vi "lorenz system.vi"(9 "Numeric":i32, 10 "array":dbl[](array[numeric])) -> (1 "z":dbl[](array[numeric]), 2 "y":dbl[](array[numeric]), 3 "x":dbl[](array[numeric]))   [LabVIEW 2019]
uses:
  <vilib>/Native 3D Graph/xcontrol/3DPC_SurfacePlot.xctl
panel:
  out "3D Graph":refnum<class "Base Datatype.lvclass">[](xcontrol)
  # "10*(y - x)\n x*(28 - z) - y\n x*y - (8/3)*z"
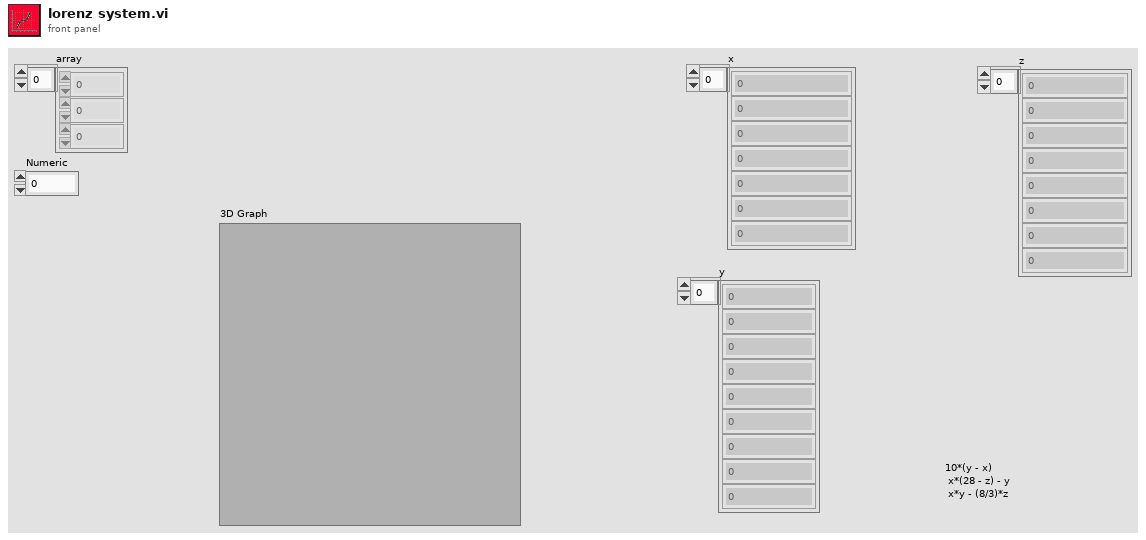
[diagram p1: front panel]
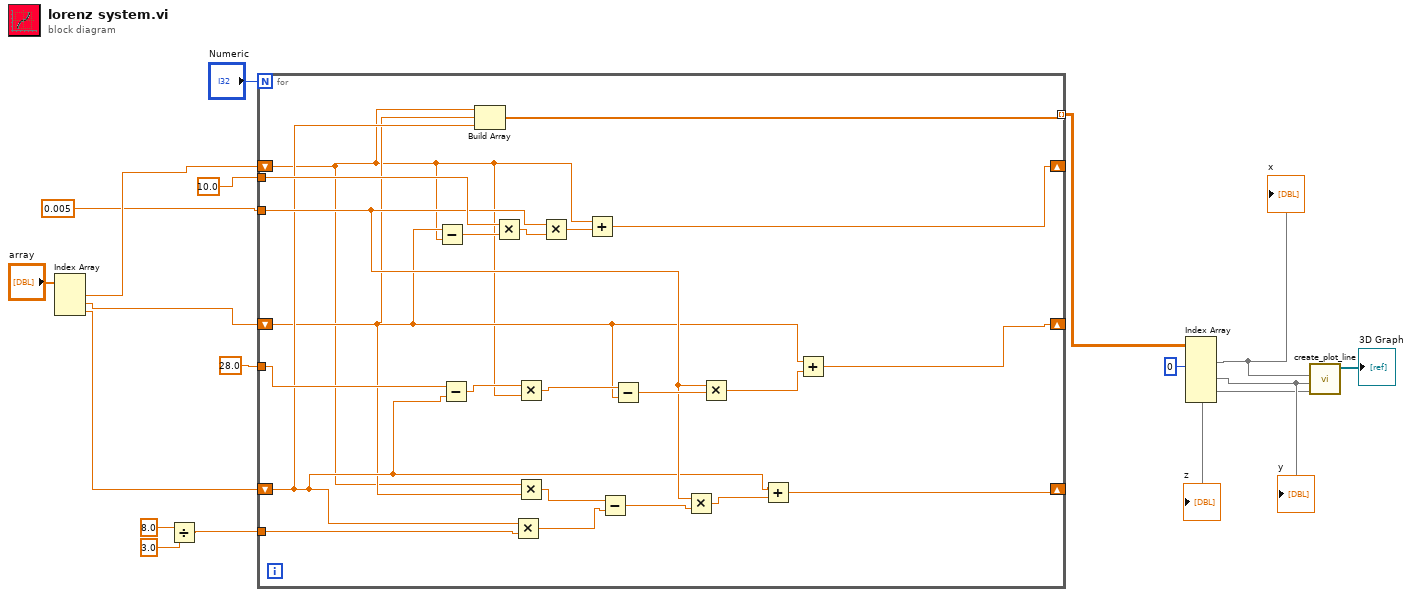
[diagram p0: block diagram]
diagram:
  n1 = Index Array(array="array") -> (element #1=w8:dbl, element #2=w11:dbl, element #3=w10:dbl)  [unwired: 3 in]
  n2 = Divide(x=8.0, y=3.0) -> (x/y=w12:dbl)
  n3 = for {
    N: "Numeric" -> [_]
    shift-right: [w35] -> _
    shift-left: w8 -> [w18]
    shift-right: [w29] -> _
    shift-left: w11 -> [w19]
    shift-right: [w22] -> _
    shift-left: w10 -> [w21]
    tunnel: 10.0 ("x") -> [w38]
    tunnel: 28.0 ("y") -> [w34]
    tunnel: 0.005 ("y") -> [w24]
    tunnel: w12 -> [w28]
    tunnel: [w20] -> w16 mode=indexing
    n4 = Subtract(x=w19, y=w18) -> (x-y=w39:dbl)
    n5 = Subtract(x=w34, y=w21) -> (x-y=w33:dbl)
    n6 = Build Array(w18, w19, w21) -> (w20:dbl[])
    n7 = Multiply(x=w38, y=w39) -> (x*y=w37:dbl)
    n8 = Multiply(x=w21, y=w28) -> (x*y=w26:dbl)
    n9 = Multiply(x=w33, y=w18) -> (x*y=w32:dbl)
    n10 = Multiply(x=w18, y=w19) -> (x*y=w27:dbl)
    n11 = Multiply(x=w24, y=w37) -> (x*y=w36:dbl)
    n12 = Add(x=w18, y=w36) -> (x+y=w35:dbl)
    n13 = Subtract(x=w27, y=w26) -> (x-y=w25:dbl)
    n14 = Subtract(x=w32, y=w19) -> (x-y=w31:dbl)
    n15 = Multiply(x=w24, y=w25) -> (x*y=w23:dbl)
    n16 = Multiply(x=w24, y=w31) -> (x*y=w30:dbl)
    n17 = Add(x=w21, y=w23) -> (x+y=w22:dbl)
    n18 = Add(x=w19, y=w30) -> (x+y=w29:dbl)
  }
  n19 = Index Array(array=w16, index (col) #1=0 ("disabled index (col)")) -> (element #1=w6:dbl[], element #2=w5:dbl[], element #3=w4:dbl[])  [unwired: 5 in]
  "x" <- w6
  "y" <- w5
  "z" <- w4
  n20 = call <vilib>:"create_plot_line.vi"("z vector"=w4, "y vector"=w5, "x vector"=w6) -> ("plots out"=→"3D Graph":refnum<class "Base Datatype.lvclass">[])  [unwired: 2 in, 6 out]
